vi "HumanExecDriveMode.vi"(4 "Enable Field Oriented Drive":bool, 5 "AutoOrientAngle":dbl, 6 "State":i32, 7 "Rotation":dbl, 8 "Right X":dbl, 9 "Right Y":dbl, 10 "Left X":dbl, 11 "Left Y":dbl) -> (0 "ExecAbsTraj":bool, 1 "AMotorDemand":dbl, 2 "YMotorDemand":dbl, 3 "XMotorDemand":dbl)   [LabVIEW 2023]
uses:
  HumanGlobal.vi
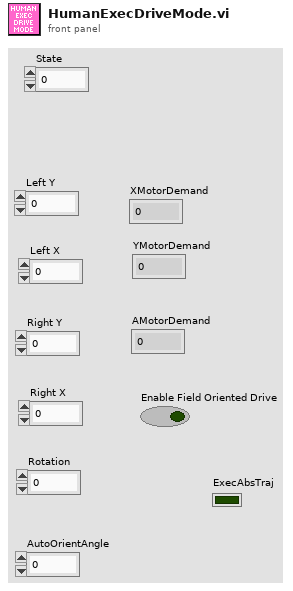
[diagram p1: front panel]
types:
  T1 = enum16{"SpeakerLeft", "SpeakerCenter", "SpeakerRight", "Amp", "Source", "StageLeft", "StageCenter", "StageRight"}
  T2 = typedef "HumanDriveModeENUM.ctl" = enum16{"0 - Normal Swerve", "1 - Auto traj  - Left Speaker", "2 - Auto traj - Center Speaker", "3 - Auto traj - Speaker Right", "4 - Auto traj - Amp", "5 - Auto traj - Source", "6 - Auto traj -  Left Stage", "7 - Auto traj - Center Stage", "8 - Auto traj - Right Stage"}
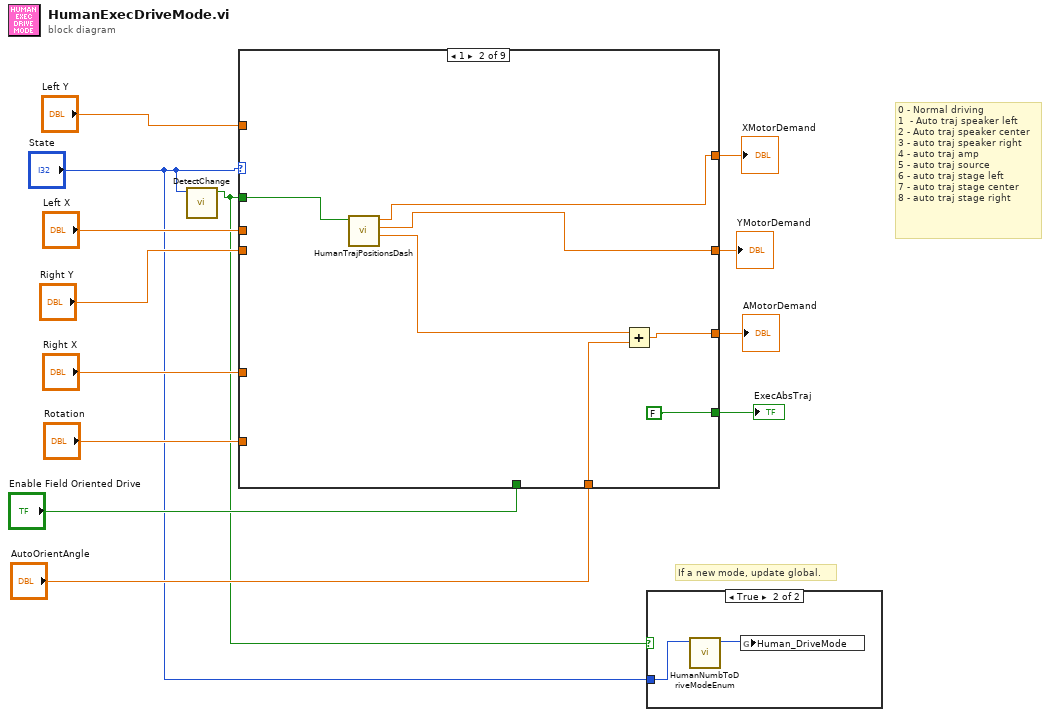
[diagram p0: block diagram]
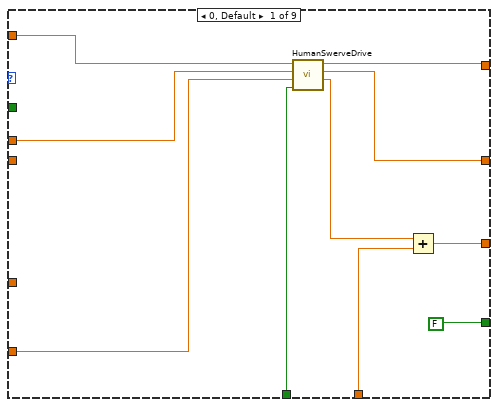
[diagram p3: hidden frame]
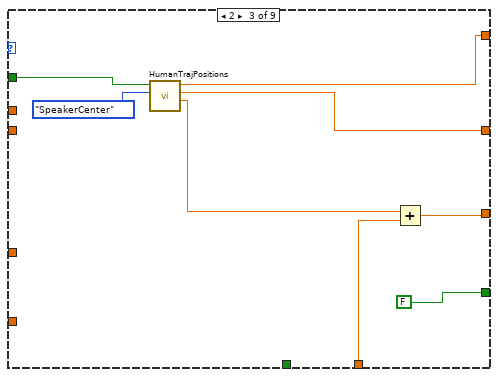
[diagram p4: hidden frame]
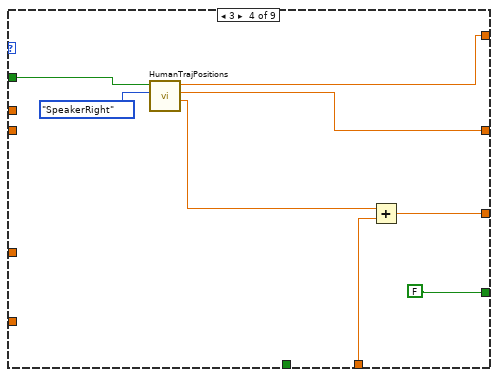
[diagram p5: hidden frame]
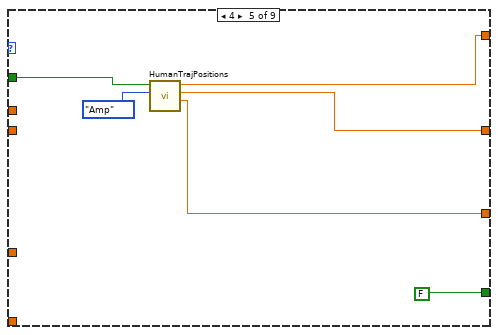
[diagram p6: hidden frame]
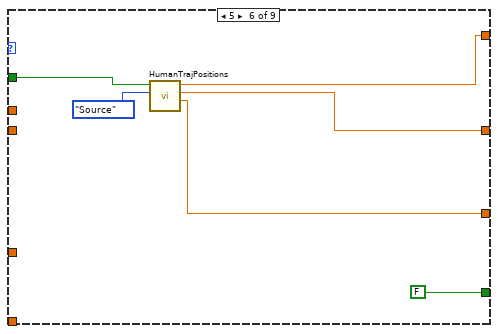
[diagram p7: hidden frame]
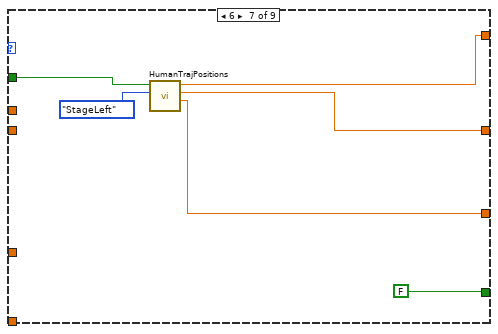
[diagram p8: hidden frame]
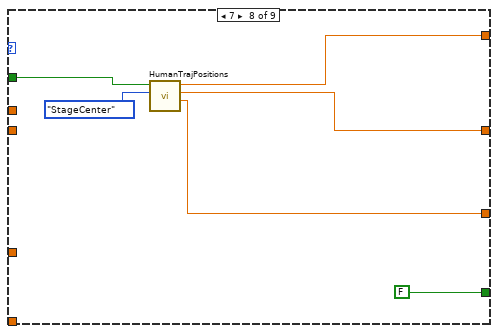
[diagram p9: hidden frame]
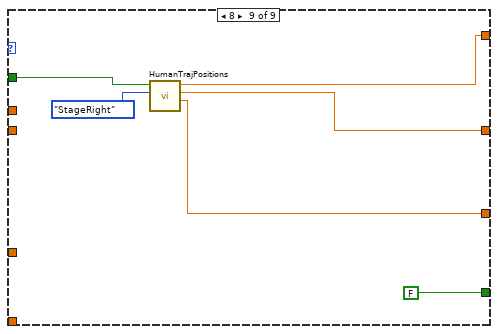
[diagram p10: hidden frame]
diagram:
  # "If a new mode, update global."
  # "0 - Normal driving\n1  - Auto traj speaker left \n2 - Auto traj speaker center\n3 - auto traj speaker right \n4 - auto traj amp\n5 - auto traj source\n6 - auto traj stage left\n7 - auto traj stage center\n8 - auto traj stage right"
  n1 = call "DetectChange.vi"("Value"="State") -> ("Changed"=w3:bool)  [unwired: 10 in]
  n2 = case shown="1" "State" {
    tunnel: "Left Y" -> [w23 _ _ _ _ _ _ _ _]
    tunnel: "Right X" -> [_ _ _ _ _ _ _ _ _]
    tunnel: [w20 w27 w37 w45 w51 w57 w63 w69 w75] -> w11
    tunnel: [w19 w26 w36 w44 w50 w56 w62 w68 w74] -> w10
    tunnel: "Right Y" -> [_ _ _ _ _ _ _ _ _]
    tunnel: w3 -> [_ w28 w38 w46 w52 w58 w64 w70 w76]
    tunnel: "Left X" -> [w22 _ _ _ _ _ _ _ _]
    tunnel: "Rotation" -> [w21 _ _ _ _ _ _ _ _]
    tunnel: [w15 w30 w33 w41 w49 w55 w61 w67 w73] -> w6
    tunnel: "Enable Field Oriented Drive" -> [w18 _ _ _ _ _ _ _ _]
    tunnel: "AutoOrientAngle" -> [w17 w29 w34 w40 _ _ _ _ _]
    tunnel: [FALSE FALSE FALSE FALSE FALSE FALSE FALSE FALSE FALSE] -> w1
    frame 0, Default {
      n3 = call "HumanSwerveDrive.vi"("Enable Field Oriented Drive"=w18, "Rotation"=w21, "Y"=w22, "X"=w23) -> ("A"=w16:dbl, "Y"=w19:dbl, "X"=w20:dbl)  [unwired: 5 in]
      n4 = Add(x=w16, y=w17) -> (x+y=w15:dbl)
    }
    frame 1 {
      n5 = call "HumanTrajPositionsDash.vi"("Init"=w28) -> ("vAngular"=w25:dbl, "vY"=w26:dbl, "vX"=w27:dbl)  [unwired: 8 in]
      n6 = Add(x=w25, y=w29) -> (x+y=w30:dbl)
    }
    frame 2 {
      n7 = call "HumanTrajPositions.vi"("FieldPos"=T1."SpeakerCenter", "Init"=w38) -> ("vAngular"=w32:dbl, "vY"=w36:dbl, "vX"=w37:dbl)  [unwired: 7 in]
      n8 = Add(x=w32, y=w34) -> (x+y=w33:dbl)
    }
    frame 3 {
      n9 = call "HumanTrajPositions.vi"("FieldPos"=T1."SpeakerRight", "Init"=w46) -> ("vAngular"=w42:dbl, "vY"=w44:dbl, "vX"=w45:dbl)  [unwired: 7 in]
      n10 = Add(x=w42, y=w40) -> (x+y=w41:dbl)
    }
    frame 4 {
      n11 = call "HumanTrajPositions.vi"("FieldPos"=T1."Amp", "Init"=w52) -> ("vAngular"=w49:dbl, "vY"=w50:dbl, "vX"=w51:dbl)  [unwired: 7 in]
    }
    frame 5 {
      n12 = call "HumanTrajPositions.vi"("FieldPos"=T1."Source", "Init"=w58) -> ("vAngular"=w55:dbl, "vY"=w56:dbl, "vX"=w57:dbl)  [unwired: 7 in]
    }
    frame 6 {
      n13 = call "HumanTrajPositions.vi"("FieldPos"=T1."StageLeft", "Init"=w64) -> ("vAngular"=w61:dbl, "vY"=w62:dbl, "vX"=w63:dbl)  [unwired: 7 in]
    }
    frame 7 {
      n14 = call "HumanTrajPositions.vi"("FieldPos"=T1."StageCenter", "Init"=w70) -> ("vAngular"=w67:dbl, "vY"=w68:dbl, "vX"=w69:dbl)  [unwired: 7 in]
    }
    frame 8 {
      n15 = call "HumanTrajPositions.vi"("FieldPos"=T1."StageRight", "Init"=w76) -> ("vAngular"=w73:dbl, "vY"=w74:dbl, "vX"=w75:dbl)  [unwired: 7 in]
    }
  }
  "XMotorDemand" <- w11
  "YMotorDemand" <- w10
  "AMotorDemand" <- w6
  "ExecAbsTraj" <- w1
  n16 = case shown="True" w3 {
    tunnel: "State" -> [_ w78]
    frame False {
    }
    frame True {
      n17 = call "HumanNumbToDriveModeEnum.vi"("DriveModeValue"=w78) -> ("DriveMode"=w77:T2)  [unwired: 10 in]
      n18 = global write "HumanGlobal.vi" "Human_DriveMode"(w77) -> ()
    }
  }
